vi "Move Labels.vi"(6 "Variant in":variant caption="变体输入", 7 "Shift Pressed?":bool caption="按下Shift？", 8 "error in (no error)":errorcluster caption="错误输入（无错误）", 10 "QD Combo Box Ref":refnum<vi> caption="快速放置组合框引用", 11 "QD Launch VI Ref":refnum<vi> caption="快速放置启动VI引用") -> (0 "error out":errorcluster caption="错误输出", 4 "Variant out":variant caption="变体输出")   [LabVIEW 2016]
doc: "重新放置各个顶层前面板和程序框图对象的可见标签/标题，保持与“工具 > 选项”中“默认标签位置”的设置一致。如同时按下[Shift]，则对（包括嵌套对象在内的）全部对象进行修改。如通过前面板激活该快捷键，则对输入和显示控件进行修改。如通过程序框图激活该快捷键，则对输入和显示控件的接线端进行修改。如激活该快捷键时，已经选定前面板/程序框图的对象，则选定对象中拥有可见标签/标题的对象会被修改。\n\n对于被修改的标签和标题，其文本调整设置也将更改为与新标签/标题位置一致。\n\n默认快捷键 - [T]"
uses:
  <vilib>/Utility/traverseref.llb/TRef TravTarget.ctl
  <vilib>/Utility/traverseref.llb/VI Scripting - Traverse.lvlib
panel:
  in  "Undo Name":string="移动标签" caption="撤消名称"
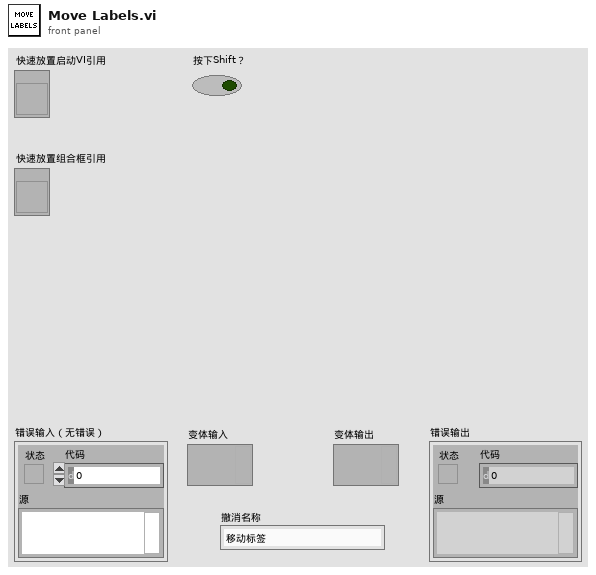
[diagram p1: front panel]
types:
  T1 = typedef "TRef TravTarget.ctl" = enum16{"FP", "BD", "Other"}
  T2 = typedef "LVRectTypeDef.ctl" = cluster{"Left":i16, "Top":i16, "Right":i16, "Bottom":i16}
  T3 = cluster{"MasterRect":T2, "Label":refnum<vi>, "f":i32}
  T4 = enum32{"None", "Size to Fit", "Arrange Horizontally", "Arrange Vertically"}
  T5 = cluster{"Bounds Rect":T2, "Label":refnum<vi>, "f":i32}
  T6 = cluster{"Bounds Rect":T2, "Label":refnum<vi>, "right-top":i32}
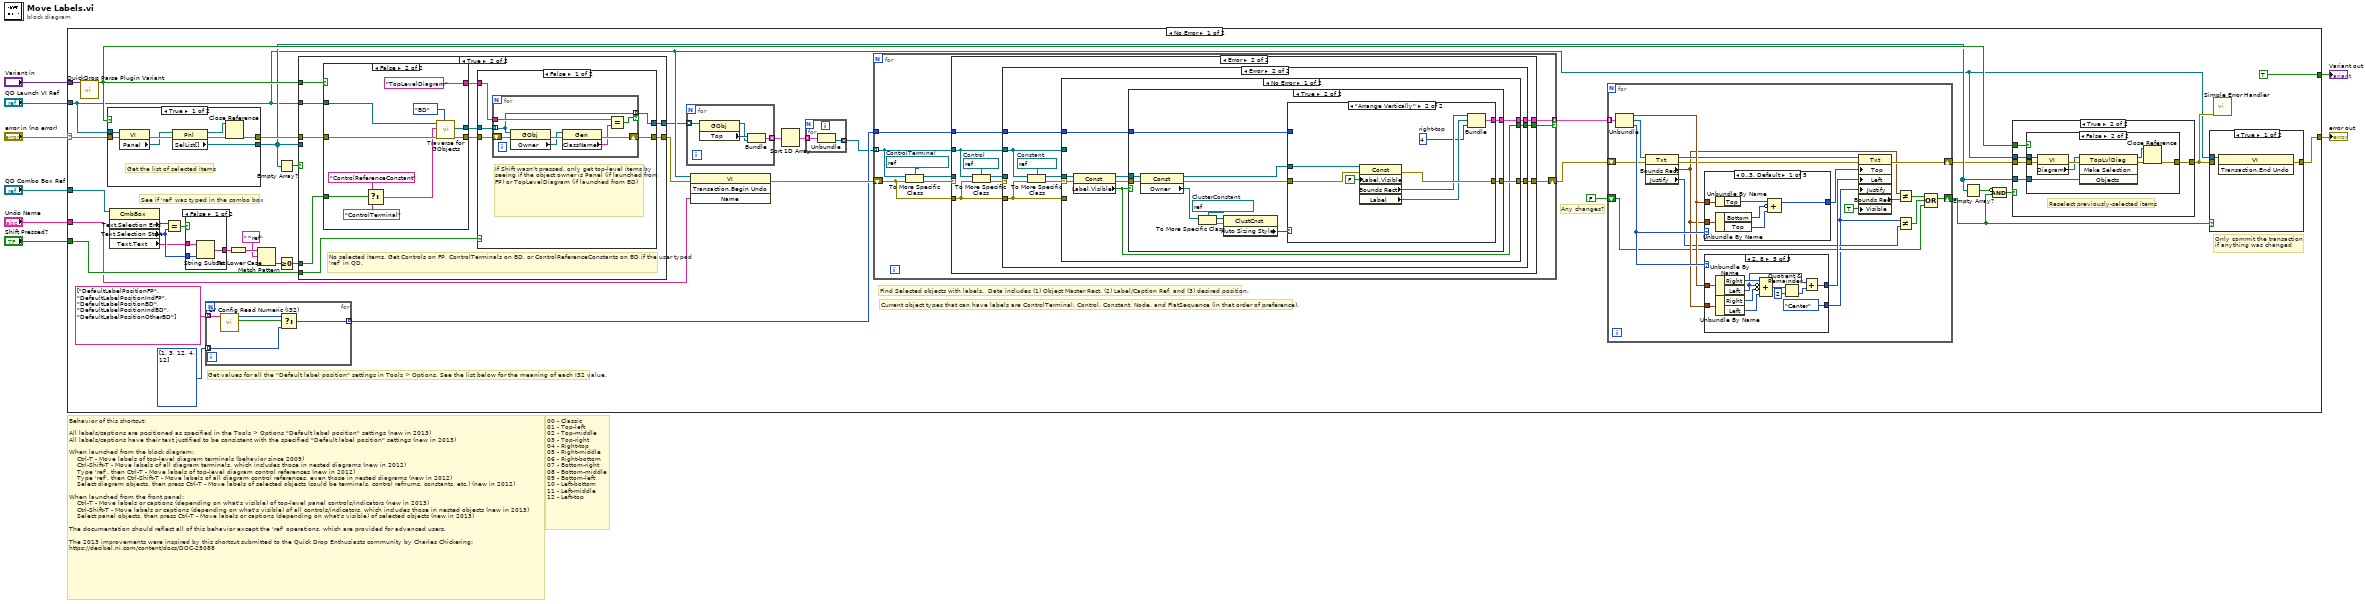
[diagram p0: block diagram]
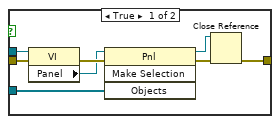
[diagram p3: hidden frame]
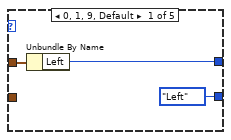
[diagram p4: hidden frame]
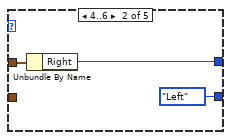
[diagram p5: hidden frame]
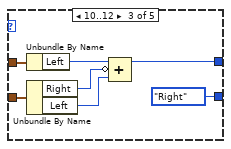
[diagram p6: hidden frame]
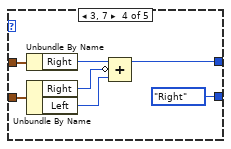
[diagram p7: hidden frame]
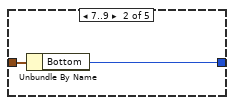
[diagram p8: hidden frame]
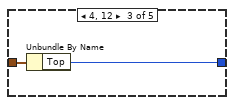
[diagram p9: hidden frame]
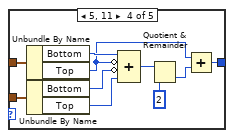
[diagram p10: hidden frame]
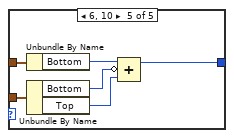
[diagram p11: hidden frame]
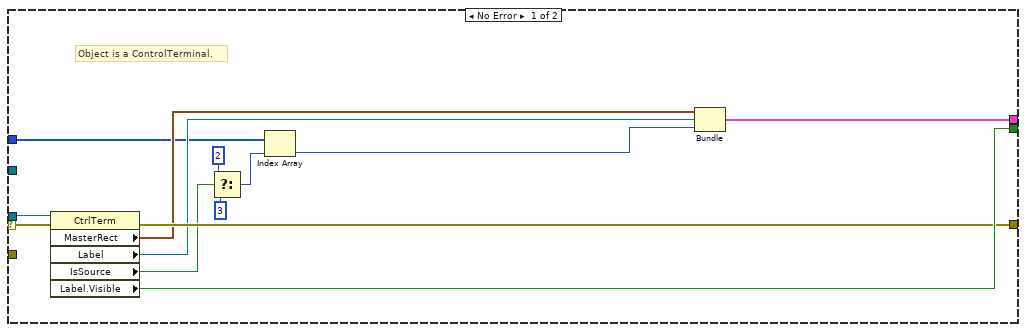
[diagram p12: hidden frame]
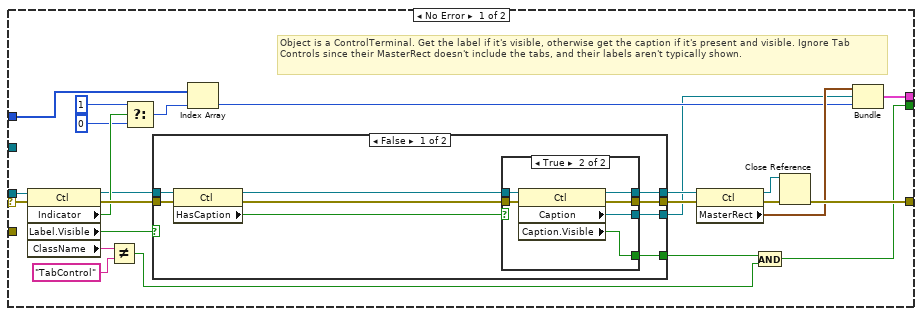
[diagram p13: hidden frame]
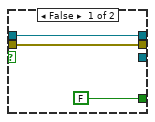
[diagram p14: hidden frame]
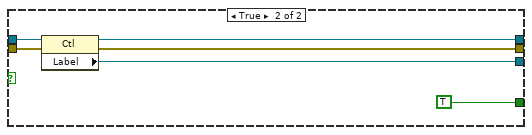
[diagram p15: hidden frame]
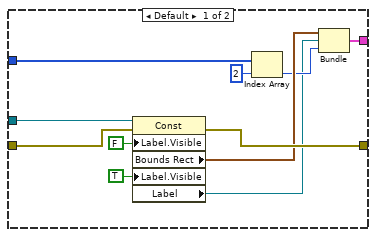
[diagram p17: hidden frame]
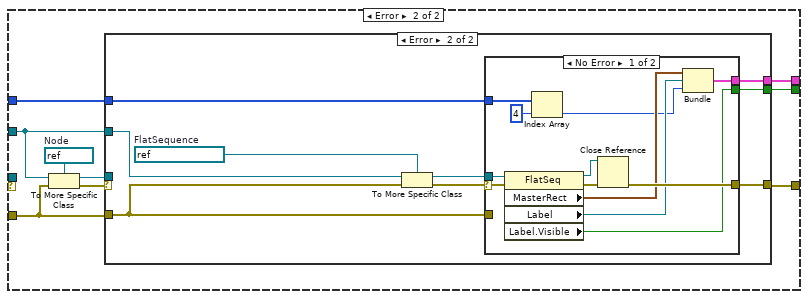
[diagram p18: hidden frame]
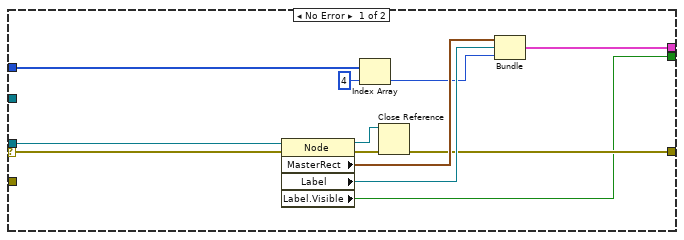
[diagram p19: hidden frame]
diagram:
  # "00 - Classic\n01 - Top-left\n02 - Top-middle\n03 - Top-right\n04 - Right-top\n05 - Right-middle\n06 - Right-bottom\n07 - Bottom-right\n08 - Bottom-middle\n09 - Bottom-left\n10 - Left-bottom\n11 - Left-middle\n12 - Left-top"
  # "Behavior of this shortcut:\n\nAll labels/captions are positioned as specified in the Tools > Options \"Default label position\" settings (new in 2013)\nAll labels/captions have their text justified to be consistent with the specified \"Default label position\" settings (new in 2013) \n\nWhen launched from the block diagram:\n    Ctrl-T - Move labels of top-level diagram terminals (behavior since 2009)\n    Ctrl-Shift-T - Move labels of all diagram terminals, which includes those in nested diagrams (new in 2012)\n    Type 'ref', then Ctrl-T - Move labels of top-level diagram control references (new in 2012)\n    Type 'ref', then Ctrl-Shift-T - Move labels of all diagram control references, even those in nested diagrams (new in 2012)\n    Select diagram objects, then press Ctrl-T - Move labels of selected objects (could be terminals, control refnums, constants, etc.) (new in 2012)\n\nWhen launched from the front panel:\n    Ctrl-T - Move labels or captions (depending on what's visible) of top-level panel controls/indicators (new in 2013)\n    Ctrl-Shift-T - Move labels or captions (depending on what's visible) of all controls/indicators, which includes those in nested objects (new in 2013)\n    Select panel objects, then press Ctrl-T - Move labels or captions (depending on what's visible) of selected objects (new in 2013)\n\nThe documentation should reflect all of this behavior except the 'ref' operations, which are provided for advanced users.\n\nThe 2013 improvements were inspired by this shortcut submitted to the Quick Drop Enthusiasts community by Charles Chickering:\nhttps://decibel.ni.com/content/docs/DOC-25088"
  n1 = case shown="No Error" "error in (no error)" {
    selector: "error in (no error)" -> [w46 w395]
    tunnel: [w22 w395] -> w7
    tunnel: "Shift Pressed?" -> [w32 _]
    tunnel: "Undo Name" -> [w15 _]
    tunnel: "QD Launch VI Ref" -> [w14 _]
    tunnel: "QD Combo Box Ref" -> [w37 _]
    tunnel: "Variant in" -> [w45 _]
    tunnel: [TRUE _] -> w1
    frame No Error {
      # "Get values for all the \"Default label position\" settings in Tools > Options. See the list below for the meaning of each I32 value."
      # "Current object types that can have labels are ControlTerminal, Control, Constant, Node, and FlatSequence (in that order of preference)."
      # "Find Selected objects with labels.  Data includes (1) Object Master Rect, (2) Label/Caption Ref, and (3) desired position."
      # "See if 'ref' was typed in the combo box"
      # "Any changes?"
      # "Only commit the transaction\nif anything was changed"
      n2 = call <vilib>:"QuickDrop Parse Plugin Variant.vi"("QDKS Variant in"=w45) -> ("QD Launch VI Panel?"=w28:bool)  [unwired: 12 in, 2 out]
      n3 = case shown="True" w28 {
        tunnel: w14 -> [w382 w390]
        tunnel: w46 -> [w381 w389]
        tunnel: [w380 w388] -> w34
        tunnel: [w379 w387] -> w26
        frame True {
          # "Get the list of selected items"
          n4 = property class="VI"(reference=w382, error in=w381) -> (error out=w386:errorcluster, "Panel"=w385:refnum<vi>)  [unwired: 1 out]
          n5 = property class="Pnl"(reference=w385, error in=w386) -> (reference out=w383:refnum<vi>, error out=w384:errorcluster, "SelList[]"=w379:refnum<vi>[])
          n6 = Close Reference(reference=w383, error in (no error)=w384) -> (error out=w380:errorcluster)
        }
        frame False {
          # "Get the list of selected items"
          n7 = property class="VI"(reference=w390, error in=w389) -> (error out=w394:errorcluster, "Diagram"=w393:refnum<vi>)  [unwired: 1 out]
          n8 = property class="TopLvlDiag"(reference=w393, error in=w394) -> (reference out=w391:refnum<vi>, error out=w392:errorcluster, "SelList[]"=w387:refnum<vi>[])
          n9 = Close Reference(reference=w391, error in (no error)=w392) -> (error out=w388:errorcluster)
        }
      }
      n10 = property on="Property Node" class="CmbBox"(reference=w37) -> ("Text.Selection End"=w44:u32, "Text.Selection Start"=w42:u32, "Text.Text"=w41:string)  [unwired: 1 in, 2 out]
      n11 = Equal?(x=w44, y=w42) -> (x = y?=w43:bool)
      n12 = case shown="False" w43 {
        tunnel: [w373 w374] -> w40
        tunnel: w42 -> [w372 _]
        tunnel: w41 -> [w371 w374]
        frame False {
          n13 = String Subset(string=w371, length (rest)=w372) -> (substring=w373:string)  [unwired: 1 out]
        }
        frame True {
        }
      }
      n14 = for {
        tunnel: string[] ["DefaultLabelPositionFP", "DefaultLabelPositionIndFP", "DefaultLabelPositionBD", "DefaultLabelPositionIndBD", "DefaultLabelPositionOtherBD"] -> [w57] mode=indexing
        tunnel: [w54] -> w13 mode=indexing
        tunnel: i32[] [1, 3, 12, 4, 12] -> [w53] mode=indexing
        n15 = call <resource>:"LV Config Read Numeric (I32).vi"("key"=w57) -> ("found?"=w56:bool, "value"=w55:i32)  [unwired: 4 in, 1 out]
        n16 = Select(t=w55, s=w56, f=w53) -> (s? t:f=w54:i32)
      }
      n17 = To Lower Case(string=w40) -> (all lower case string=w39:string)
      n18 = Match Pattern(string=w39, regular expression="^ref") -> (offset past match=w36:i32)  [unwired: 1 in, 3 out]
      n19 = Empty Array?(array=w26) -> (empty?=w35:bool)
      n20 = Greater Or Equal To 0?(x=w36) -> (x >= 0?=w33:bool)
      n21 = case shown="True" w35 {
        tunnel: w26 -> [w328 _]
        tunnel: w34 -> [w327 w337]
        tunnel: [w328 w330] -> w12
        tunnel: w28 -> [_ w338]
        tunnel: w33 -> [_ w335]
        tunnel: w14 -> [_ w336]
        tunnel: w32 -> [_ w332]
        tunnel: [w327 w331] -> w16
        frame False {
          # "There were selected items. Only operate on those."
        }
        frame True {
          # "No selected items. Get Controls on FP, ControlTerminals on BD, or ControlReferenceConstants on BD if the user typed 'ref' in QD."
          n22 = case shown="False" w338 {
            tunnel: w337 -> [w360 w370]
            tunnel: w336 -> [w359 w369]
            tunnel: [w356 w367] -> w334
            tunnel: [w355 w366] -> w333
            tunnel: ["Panel" "TopLevelDiagram"] -> w329
            tunnel: w335 -> [_ w364]
            frame True {
              n23 = call <vilib>:"Traverse for GObjects.vi"("Traverse Target"=TRef_TravTarget."FP", "error in (no error)"=w360, "Class Name"="Control", "VI Refnum"=w359) -> ("error out"=w356:errorcluster, "References"=w355:refnum<vi>[])  [unwired: 4 in, 2 out]
            }
            frame False {
              n24 = Select(t="ControlReferenceConstant", s=w364, f="ControlTerminal") -> (s? t:f=w363:string)
              n25 = call <vilib>:"Traverse for GObjects.vi"("Traverse Target"=TRef_TravTarget."BD", "error in (no error)"=w370, "Class Name"=w363, "VI Refnum"=w369) -> ("error out"=w367:errorcluster, "References"=w366:refnum<vi>[])  [unwired: 4 in, 2 out]
            }
          }
          n26 = case shown="False" w332 {
            tunnel: w334 -> [w343 w353]
            tunnel: w333 -> [w342 w352]
            tunnel: [w340 w353] -> w331
            tunnel: [w339 w352] -> w330
            tunnel: w329 -> [w341 _]
            frame False {
              # "If Shift wasn't pressed, only get top-level items by seeing if the object owner is Panel (if launched from FP) or TopLevelDiagram (if launched from BD)"
              n27 = for {
                shift-right: [w348] -> w340
                shift-left: w343 -> [w351]
                tunnel: w342 -> [w345] mode=indexing
                tunnel: w341 -> [w346]
                tunnel: [w345] -> w339 mode=indexing if=w344
                n28 = property class="GObj"(reference=w345, error in=w351) -> (error out=w350:errorcluster, "Owner"=w349:refnum<vi>)  [unwired: 1 out]
                n29 = property class="Gen"(reference=w349, error in=w350) -> (error out=w348:errorcluster, "ClassName"=w347:string)  [unwired: 1 out]
                n30 = Equal?(x=w346, y=w347) -> (x = y?=w344:bool)
              }
            }
            frame True {
            }
          }
        }
      }
      n31 = for {
        tunnel: w12 -> [w52] mode=indexing
        tunnel: [w49] -> w11 mode=indexing
        n32 = property class="GObj"(reference=w52) -> (reference out=w50:refnum<vi>, "Top"=w51:i32)  [unwired: 1 in, 1 out]
        n33 = Bundle("Top"=w51, w50) -> (w49:cluster{"Top":i32, refnum<vi>})  [unwired: 1 in]
      }
      n34 = invoke class="VI" method="Transaction.Begin Undo"(reference=w14, error in=w16, "Name"=w15) -> (error out=w17:errorcluster)  [unwired: 1 in, 3 out]
      n35 = Sort 1D Array(array=w11) -> (sorted array=w10:cluster{"Top":i32, refnum<vi>}[])
      n36 = for {
        tunnel: w10 -> [w48] mode=indexing
        tunnel: [w47] -> w9 mode=indexing
        n37 = Unbundle(w48) -> (w47:refnum<vi>)  [unwired: 1 out]
      }
      n38 = for {
        shift-right: [w164] -> w18
        shift-left: w17 -> [w156]
        tunnel: w9 -> [w162] mode=indexing
        tunnel: [w163] -> w31 mode=indexing if=w158
        tunnel: w13 -> [w157]
        w159 = refnum<vi> refnum  # ControlTerminal
        n39 = To More Specific Class(target class=w159, reference=w162, error in=w156) -> (specific class reference=w160:refnum<vi>, error out=w161:errorcluster)
        n40 = case shown="Error" w161 {
          selector: w161 -> [w176 _]
          tunnel: [w174 w183] -> w164
          tunnel: w162 -> [_ w182]
          tunnel: [w171 w181] -> w163
          tunnel: w160 -> [w177 _]
          tunnel: [w175 w179] -> w158
          tunnel: w157 -> [w170 w180]
          tunnel: w156 -> [_ w178]
          frame No Error {
            # "Object is a ControlTerminal."
            n41 = property class="CtrlTerm"(reference=w177, error in=w176) -> (error out=w174:errorcluster, "MasterRect"=w173:T2, "Label"=w172:refnum<vi>, "IsSource"=w169:bool, "Label.Visible"=w175:bool)  [unwired: 1 out]
            n42 = Select(t=2, s=w169, f=3) -> (s? t:f=w166:i32)
            n43 = Index Array(array=w170, index=w166) -> (element=w165:i32)
            n44 = Bundle("MasterRect"=w173, "Label"=w172, "f"=w165) -> (w171:T3)  [unwired: 1 in]
          }
          frame Error {
            w186 = refnum<vi> refnum  # Control
            n45 = To More Specific Class(target class=w186, reference=w182, error in=w178) -> (specific class reference=w185:refnum<vi>, error out=w184:errorcluster)
            n46 = case shown="Error" w184 {
              selector: w184 -> [w210 _]
              tunnel: w185 -> [w203 _]
              tunnel: [w207 w239] -> w183
              tunnel: w178 -> [_ w240]
              tunnel: w182 -> [_ w238]
              tunnel: [w205 w237] -> w181
              tunnel: w180 -> [w191 w235]
              tunnel: [w188 w236] -> w179
              frame No Error {
                # "Object is a ControlTerminal. Get the label if it's visible, otherwise get the caption if it's present and visible. Ignore Tab Controls since their MasterRect doesn't include the tabs, and their labels aren't typically shown."
                n47 = property class="Ctl"(reference=w203, error in=w210) -> (reference out=w196:refnum<vi>, error out=w204:errorcluster, "Indicator"=w202:bool, "Label.Visible"=w194:bool, "ClassName"=w190:string)
                n48 = Not Equal?(x=w190, y="TabControl") -> (x != y?=w187:bool)
                n49 = Select(t=1, s=w202, f=0) -> (s? t:f=w199:i32)
                n50 = case shown="False" w194 {
                  tunnel: w204 -> [w219 w234]
                  tunnel: [w216 w231] -> w197
                  tunnel: w196 -> [w217 w233]
                  tunnel: [w214 w232] -> w195
                  tunnel: [w212 w230] -> w193
                  tunnel: [w211 TRUE] -> w192
                  frame False {
                    n51 = property class="Ctl"(reference=w217, error in=w219) -> (reference out=w215:refnum<vi>, error out=w218:errorcluster, "HasCaption"=w213:bool)
                    n52 = case shown="True" w213 {
                      tunnel: w218 -> [w221 w228]
                      tunnel: [w221 w227] -> w216
                      tunnel: w215 -> [w222 w226]
                      tunnel: [w222 w225] -> w214
                      tunnel: [_ w224] -> w212
                      tunnel: [FALSE w223] -> w211
                      frame False {
                      }
                      frame True {
                        n53 = property class="Ctl"(reference=w226, error in=w228) -> (reference out=w225:refnum<vi>, error out=w227:errorcluster, "Caption"=w224:refnum<vi>, "Caption.Visible"=w223:bool)
                      }
                    }
                  }
                  frame True {
                    n54 = property class="Ctl"(reference=w233, error in=w234) -> (reference out=w232:refnum<vi>, error out=w231:errorcluster, "Label"=w230:refnum<vi>)
                  }
                }
                n55 = Index Array(array=w191, index=w199) -> (element=w198:i32)
                n56 = property class="Ctl"(reference=w195, error in=w197) -> (reference out=w208:refnum<vi>, error out=w209:errorcluster, "MasterRect"=w206:T2)
                n57 = And(x=w192, y=w187) -> (x .and. y?=w188:bool)
                n58 = Close Reference(reference=w208, error in (no error)=w209) -> (error out=w207:errorcluster)
                n59 = Bundle("MasterRect"=w206, "Label"=w193, "f"=w198) -> (w205:T3)  [unwired: 1 in]
              }
              frame Error {
                w243 = refnum<vi> refnum  # Constant
                n60 = To More Specific Class(target class=w243, reference=w238, error in=w240) -> (specific class reference=w241:refnum<vi>, error out=w242:errorcluster)
                n61 = case shown="No Error" w242 {
                  selector: w242 -> [w251 _]
                  tunnel: w240 -> [_ w288]
                  tunnel: w241 -> [w246 _]
                  tunnel: [w250 w289] -> w239
                  tunnel: w238 -> [_ w287]
                  tunnel: [w249 w286] -> w237
                  tunnel: [w244 w285] -> w236
                  tunnel: w235 -> [w248 w284]
                  frame No Error {
                    n62 = property class="Const"(reference=w246, error in=w251) -> (reference out=w245:refnum<vi>, error out=w247:errorcluster, "Label.Visible"=w244:bool)
                    n63 = case shown="True" w244 {
                      tunnel: [w252 w264] -> w250
                      tunnel: [_ w263] -> w249
                      tunnel: w248 -> [_ w262]
                      tunnel: w247 -> [w252 w261]
                      tunnel: w245 -> [_ w259]
                      frame False {
                      }
                      frame True {
                        w256 = refnum<vi> refnum  # ClusterConstant
                        n64 = property class="Const"(reference=w259, error in=w261) -> (reference out=w258:refnum<vi>, error out=w260:errorcluster, "Owner"=w257:refnum<vi>)
                        n65 = To More Specific Class(target class=w256, reference=w257) -> (specific class reference=w254:refnum<vi>, error out=w255:errorcluster)  [unwired: 1 in]
                        n66 = property class="ClustCnst"(reference=w254, error in=w255) -> ("Auto Sizing Style"=w253:T4)  [unwired: 2 out]
                        n67 = case shown="\"Arrange Vertically\"" w253 {
                          tunnel: [w275 w283] -> w264
                          tunnel: [w273 w281] -> w263
                          tunnel: w262 -> [w272 _]
                          tunnel: w260 -> [w266 w278]
                          tunnel: w258 -> [w265 w277]
                          frame Default {
                            n68 = property class="Const"(reference=w265, error in=w266, "Label.Visible"=FALSE, "Label.Visible"=TRUE) -> (error out=w275:errorcluster, "Bounds Rect"=w274:T2, "Label"=w269:refnum<vi>)  [unwired: 1 out]
                            n69 = Index Array(array=w272, index=2) -> (element=w270:i32)
                            n70 = Bundle("Bounds Rect"=w274, "Label"=w269, "f"=w270) -> (w273:T5)  [unwired: 1 in]
                          }
                          frame "Arrange Vertically" {
                            w276 = 4  # right-top
                            n71 = property class="Const"(reference=w277, error in=w278, "Label.Visible"=FALSE) -> (error out=w283:errorcluster, "Bounds Rect"=w282:T2, "Label"=w280:refnum<vi>)  [unwired: 1 out]
                            n72 = Bundle("Bounds Rect"=w282, "Label"=w280, "right-top"=w276) -> (w281:T6)  [unwired: 1 in]
                          }
                        }
                      }
                    }
                  }
                  frame Error {
                    w292 = refnum<vi> refnum  # Node
                    n73 = To More Specific Class(target class=w292, reference=w287, error in=w288) -> (specific class reference=w290:refnum<vi>, error out=w291:errorcluster)
                    n74 = case shown="Error" w291 {
                      selector: w291 -> [w304 _]
                      tunnel: w290 -> [w302 _]
                      tunnel: [w299 w308] -> w289
                      tunnel: w288 -> [_ w309]
                      tunnel: w287 -> [_ w312]
                      tunnel: [w297 w307] -> w286
                      tunnel: [w296 w305] -> w285
                      tunnel: w284 -> [w295 w306]
                      frame No Error {
                        n75 = property class="Node"(reference=w302, error in=w304) -> (reference out=w298:refnum<vi>, error out=w303:errorcluster, "MasterRect"=w301:T2, "Label"=w300:refnum<vi>, "Label.Visible"=w296:bool)
                        n76 = Index Array(array=w295, index=4) -> (element=w293:i32)
                        n77 = Close Reference(reference=w298, error in (no error)=w303) -> (error out=w299:errorcluster)
                        n78 = Bundle("MasterRect"=w301, "Label"=w300, "f"=w293) -> (w297:T3)  [unwired: 1 in]
                      }
                      frame Error {
                        w313 = refnum<vi> refnum  # FlatSequence
                        n79 = To More Specific Class(target class=w313, reference=w312, error in=w309) -> (specific class reference=w310:refnum<vi>, error out=w311:errorcluster)
                        n80 = case shown="No Error" w311 {
                          selector: w311 -> [w325 _]
                          tunnel: w310 -> [w324 _]
                          tunnel: w309 -> [_ w326]
                          tunnel: [w321 w326] -> w308
                          tunnel: [w318 _] -> w307
                          tunnel: w306 -> [w317 _]
                          tunnel: [w314 _] -> w305
                          frame No Error {
                            n81 = property class="FlatSeq"(reference=w324, error in=w325) -> (reference out=w322:refnum<vi>, error out=w323:errorcluster, "MasterRect"=w320:T2, "Label"=w319:refnum<vi>, "Label.Visible"=w314:bool)
                            n82 = Index Array(array=w317, index=4) -> (element=w315:i32)
                            n83 = Close Reference(reference=w322, error in (no error)=w323) -> (error out=w321:errorcluster)
                            n84 = Bundle("MasterRect"=w320, "Label"=w319, "f"=w315) -> (w318:T3)  [unwired: 1 in]
                          }
                          frame Error {
                          }
                        }
                      }
                    }
                  }
                }
              }
            }
          }
        }
      }
      n85 = for {
        tunnel: w31 -> [w98] mode=indexing
        shift-right: [w95] -> w24
        shift-left: w18 -> [w93]
        shift-right: [w82] -> w23
        shift-left: FALSE -> [w83]
        n86 = Unbundle(w98) -> ("MasterRect"=w96:T2, "Label"=w94:refnum<vi>, "f"=w97:i32)
        n87 = property class="Txt"(reference=w94, error in=w93) -> (reference out=w92:refnum<vi>, error out=w90:errorcluster, "Bounds Rect"=w88:T2, "Justify"=w85:enum16{"Left", "Center", "Right"})
        n88 = case shown="0..3, Default" w97 {
          tunnel: w96 -> [w135 w137 w139 w149 w155]
          tunnel: w88 -> [w134 _ _ w148 w154]
          tunnel: [w130 w136 w138 w144 w150] -> w91
          frame 0..3, Default {
            n89 = Unbundle By Name(w135) -> ("Top"=w133:i16)
            n90 = Unbundle By Name(w134) -> ("Bottom"=w132:i16, "Top"=w131:i16)
            n91 = Compound Arithmetic op=ADD(w133, invert w132, w131) -> (w130:i16)
          }
          frame 7..9 {
            n92 = Unbundle By Name(w137) -> ("Bottom"=w136:i16)
          }
          frame 4, 12 {
            n93 = Unbundle By Name(w139) -> ("Top"=w138:i16)
          }
          frame 5, 11 {
            n94 = Unbundle By Name(w149) -> ("Bottom"=w143:i16, "Top"=w142:i16)
            n95 = Unbundle By Name(w148) -> ("Bottom"=w147:i16, "Top"=w146:i16)
            n96 = Compound Arithmetic op=ADD(w143, invert w142, invert w147, w146) -> (w141:i16)
            n97 = Quotient & Remainder(x=w141, y=i16 2) -> (floor(x/y)=w145:i16)  [unwired: 1 out]
            n98 = Add(x=w142, y=w145) -> (x+y=w144:i16)
          }
          frame 6, 10 {
            n99 = Unbundle By Name(w155) -> ("Bottom"=w153:i16)
            n100 = Unbundle By Name(w154) -> ("Bottom"=w152:i16, "Top"=w151:i16)
            n101 = Compound Arithmetic op=ADD(w153, invert w152, w151) -> (w150:i16)
          }
        }
        n102 = case shown="2, 8" w97 {
          tunnel: w96 -> [w101 w104 w111 w118 w127]
          tunnel: w88 -> [_ _ w109 w116 w126]
          tunnel: [w100 w103 w106 w113 w123] -> w86
          tunnel: [enum16{"Left", "Center", "Right"}."Left" ("Justification") enum16{"Left", "Center", "Right"}."Left" ("Justification") enum16{"Left", "Center", "Right"}."Right" ("Justification") enum16{"Left", "Center", "Right"}."Right" ("Justification") enum16{"Left", "Center", "Right"}."Center" ("Justification")] -> w81
          frame 0, 1, 9, Default {
            n103 = Unbundle By Name(w101) -> ("Left"=w100:i16)
          }
          frame 4..6 {
            n104 = Unbundle By Name(w104) -> ("Right"=w103:i16)
          }
          frame 10..12 {
            n105 = Unbundle By Name(w111) -> ("Left"=w110:i16)
            n106 = Unbundle By Name(w109) -> ("Right"=w108:i16, "Left"=w107:i16)
            n107 = Compound Arithmetic op=ADD(w110, invert w108, w107) -> (w106:i16)
          }
          frame 3, 7 {
            n108 = Unbundle By Name(w118) -> ("Right"=w117:i16)
            n109 = Unbundle By Name(w116) -> ("Right"=w115:i16, "Left"=w114:i16)
            n110 = Compound Arithmetic op=ADD(w117, invert w115, w114) -> (w113:i16)
          }
          frame 2, 8 {
            n111 = Unbundle By Name(w127) -> ("Right"=w125:i16, "Left"=w122:i16)
            n112 = Unbundle By Name(w126) -> ("Right"=w128:i16, "Left"=w129:i16)
            n113 = Compound Arithmetic op=ADD(w125, invert w122, invert w128, w129) -> (w120:i16)
            n114 = Quotient & Remainder(x=w120, y=i16 2) -> (floor(x/y)=w124:i16)  [unwired: 1 out]
            n115 = Add(x=w122, y=w124) -> (x+y=w123:i16)
          }
        }
        n116 = property class="Txt"(reference=w92, error in=w90, "Top"=w91, "Left"=w86, "Justify"=w81, "Visible"=TRUE) -> (error out=w95:errorcluster, "Bounds Rect"=w89:T2)  [unwired: 1 out]
        n117 = Not Equal?(x=w88, y=w89) -> (x != y?=w87:bool)
        n118 = Not Equal?(x=w81, y=w85) -> (x != y?=w84:bool)
        n119 = Compound Arithmetic op=OR(w87, w84, w83) -> (w82:bool)
      }
      n120 = Empty Array?(array=w26) -> (empty?=w25:bool)
      n121 = Compound Arithmetic op=AND(invert w25, w23) -> (w27:bool)
      n122 = case shown="True" w27 {
        tunnel: w24 -> [w58 w63]
        tunnel: [w58 w62] -> w19
        tunnel: w14 -> [_ w61]
        tunnel: w28 -> [_ w60]
        tunnel: w26 -> [_ w59]
        frame False {
          # "No changes, and/or no selected items originally"
        }
        frame True {
          # "Reselect previously-selected items"
          n123 = case shown="False" w60 {
            tunnel: w61 -> [w67 w75]
            tunnel: w63 -> [w66 w74]
            tunnel: [w65 w73] -> w62
            tunnel: w59 -> [w64 w72]
            frame True {
              n124 = property class="VI"(reference=w67, error in=w66) -> (error out=w71:errorcluster, "Panel"=w70:refnum<vi>)  [unwired: 1 out]
              n125 = invoke class="Pnl" method="Make Selection"(reference=w70, error in=w71, "Objects"=w64) -> (reference out=w68:refnum<vi>, error out=w69:errorcluster)  [unwired: 1 in, 2 out]
              n126 = Close Reference(reference=w68, error in (no error)=w69) -> (error out=w65:errorcluster)
            }
            frame False {
              n127 = property class="VI"(reference=w75, error in=w74) -> (error out=w79:errorcluster, "Diagram"=w78:refnum<vi>)  [unwired: 1 out]
              n128 = invoke class="TopLvlDiag" method="Make Selection"(reference=w78, error in=w79, "Objects"=w72) -> (reference out=w76:refnum<vi>, error out=w77:errorcluster)  [unwired: 1 in, 2 out]
              n129 = Close Reference(reference=w76, error in (no error)=w77) -> (error out=w73:errorcluster)
            }
          }
        }
      }
      n130 = case shown="True" w23 {
        tunnel: w14 -> [w376 w378]
        tunnel: [w375 w377] -> w22
        tunnel: w19 -> [_ _]
        frame True {
          n131 = invoke class="VI" method="Transaction.End Undo"(reference=w376) -> (error out=w375:errorcluster)  [unwired: 2 in, 2 out]
        }
        frame False {
          n132 = invoke class="VI" method="Transaction.Fail"(reference=w378) -> (error out=w377:errorcluster)  [unwired: 2 in, 2 out]
        }
      }
      n133 = call <vilib>:"Simple Error Handler.vi"("error in (no error)"=w19) -> ()  [unwired: 4 in, 5 out]
    }
    frame Error {
    }
  }
  "error out" <- w7
  "Variant out" <- w1
